vi "Add DataRow to DataTable by Values.vi"(8 "错误输入（无错误）":errorcluster, 10 "values":refnum<k24>[](array[refnum]), 11 "DataTable":refnum<k24>) -> (0 "错误输出":errorcluster, 3 "DataTable":refnum<k24>)   [LabVIEW 2012, in "DataGridView.lvlib"]
uses:
  DataGridView.lvlib
  System.Data
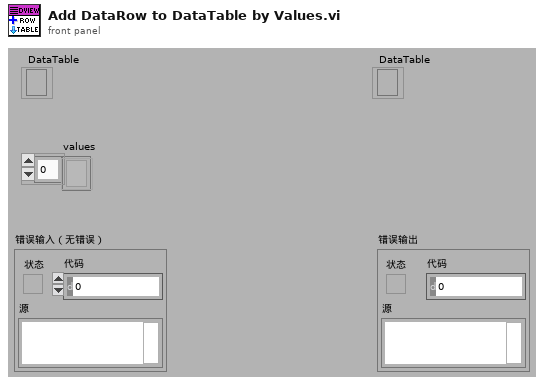
[diagram p1: front panel]
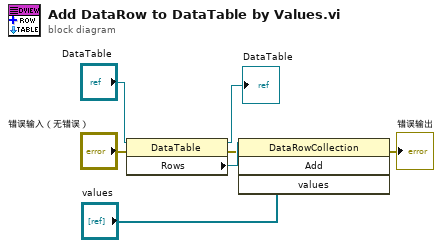
[diagram p0: block diagram]
diagram:
  n1 = property class="DataTable"(reference="DataTable", error in="错误输入（无错误）") -> (reference out=→"DataTable":refnum<k24>, error out=w2:errorcluster, "Rows"=w6:refnum<k24>)
  n2 = invoke class="DataRowCollection" method="Add"(reference=w6, error in=w2, "values"="values") -> (error out=→"错误输出":errorcluster)  [unwired: 1 in, 3 out]
